vi "QC_RunInformation.vi"() -> ()   [LabVIEW 2013]
panel:
  out "LocalConfiguration":T1={"Institute"="", "Manufacturers"=[], "Devices"=[], "Serialnumbers Lookup DB"="", "Data directory"="", "Backup & screenshot directory"="", "List of known users"=[], "Measurement switch not used"=TRUE, "Measurement Switch"="Pickering Matrix", "DUT Switch"="Keithley 3706A"}
  in  "Run info":T2={"Sensor Serial No.:"="", "Wafer Serial No.:"="", "Batch:"="", "Manufacturer:"="Hamamatsu", "Device Category:"="ATLAS18SS", "Database Serial No.:"="", "Date Initiated:"="", "Time Initiated:"="", "Test"="IV", "Instruments used:"="", "Probeplan used:"="", "End of Run comment:"="", "User:"=""}
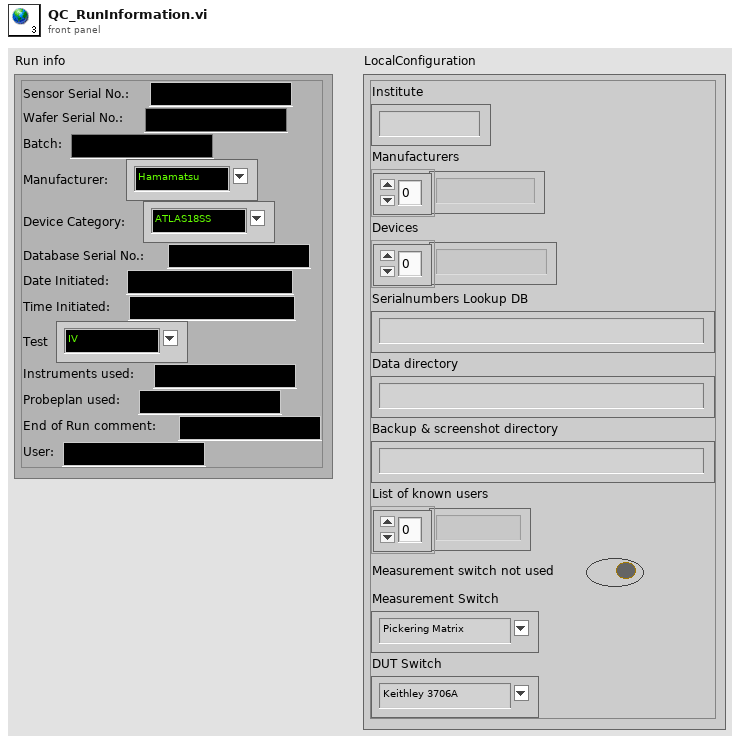
[diagram p1: front panel]
types:
  T1 = cluster{"Institute":string, "Manufacturers":string[], "Devices":string[], "Serialnumbers Lookup DB":string, "Data directory":string, "Backup & screenshot directory":string, "List of known users":string[], "Measurement switch not used":bool, "Measurement Switch":string, "DUT Switch":string}
  T2 = cluster{"Sensor Serial No.:":string, "Wafer Serial No.:":string, "Batch:":string, "Manufacturer:":string, "Device Category:":string, "Database Serial No.:":string, "Date Initiated:":string, "Time Initiated:":string, "Test":string, "Instruments used:":string, "Probeplan used:":string, "End of Run comment:":string, "User:":string}
diagram:
